vi "destroy.vi"(8 "error in (no error)":errorcluster, 11 "BoolUserEventStopMechanism In":refnum<class "BoolUserEventStopMechanism.lvclass">) -> (0 "error out":errorcluster, 3 "BoolUserEventStopMechanism Out":refnum<class "BoolUserEventStopMechanism.lvclass">)   [LabVIEW 2023, in "TLC_Daemon.lvlib" / "BoolUserEventStopMechanism.lvclass"]
doc: "Destroy procedure\n_____________________________________\nTLC Daemon 1.0.0.2\nCopyright (c) 2026 Andrea Cadei"
uses:
  BoolUserEventStopMechanism.lvclass
  BoolUserEventStopMechanism.lvclass/BoolUserEventStopMechanism.ctl
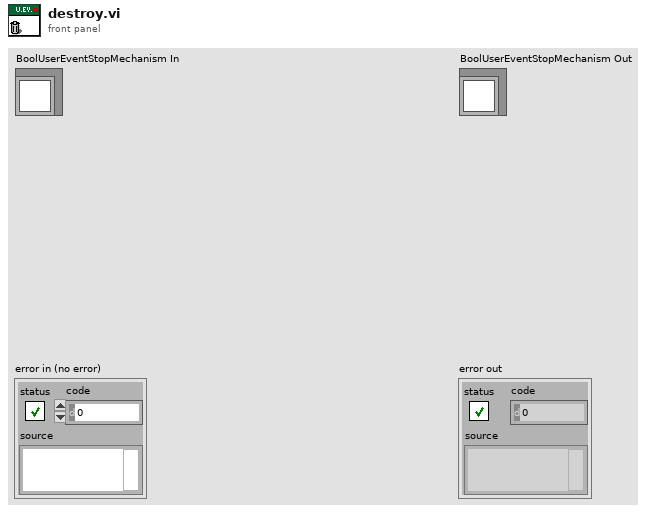
[diagram p1: front panel]
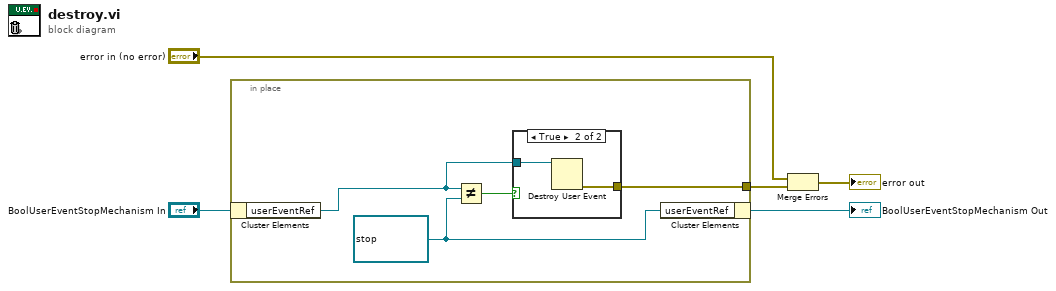
[diagram p0: block diagram]
diagram:
  n1 = in-place {
    in-place-border: [w6] -> w2
    w9 = refnum<user-event> refnum ("userEventRef")
    n2 = in-place-cluster #1("BoolUserEventStopMechanism In") -> ("userEventRef"=w7:refnum<user-event>)
    n3 = Not Equal?(x=w7, y=w9) -> (x != y?=w8:bool)
    n4 = case shown="True" w8 {
      tunnel: w7 -> [_ w11]
      tunnel: [_ w10] -> w6
      frame False {
      }
      frame True {
        n5 = Destroy User Event(user event=w11) -> (error out=w10:errorcluster)  [unwired: 1 in]
      }
    }
    n6 = in-place-cluster #1("userEventRef"=w9) -> (→"BoolUserEventStopMechanism Out":refnum<class "BoolUserEventStopMechanism.lvclass">)
  }
  n7 = Merge Errors("error in (no error)", w2) -> (→"error out":errorcluster)
